vi "padé.vi"(2 "Retardo padé":dbl, 3 "Den":dbl[](array[numeric]), 4 "Num":dbl[](array[numeric])) -> (0 "DEN":dbl[](array[numeric]), 1 "NUM":dbl[](array[numeric]))   [LabVIEW 2019]
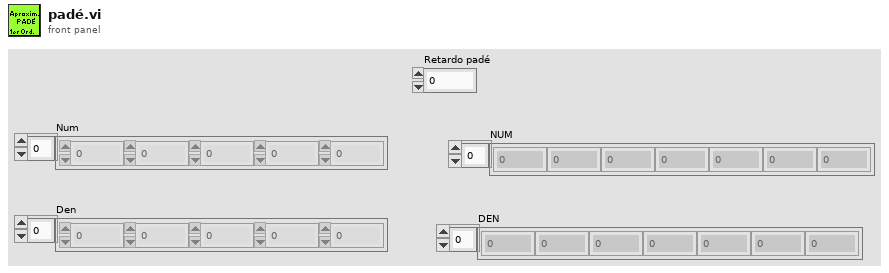
[diagram p1: front panel]
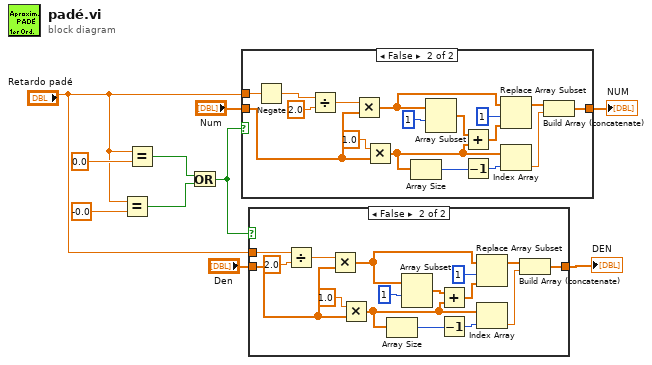
[diagram p0: block diagram]
diagram:
  n1 = Equal?(x="Retardo padé", y=-0.0) -> (x = y?=w7:bool)
  n2 = Equal?(x="Retardo padé", y=0.0) -> (x = y?=w8:bool)
  n3 = Or(x=w8, y=w7) -> (x .or. y?=w2:bool)
  n4 = case shown="False" w2 {
    tunnel: "Retardo padé" -> [_ w15]
    tunnel: [w11 w13] -> w4
    tunnel: "Num" -> [w11 w12]
    frame True {
    }
    frame False {
      n5 = Negate(x=w15) -> (-x=w14:dbl)
      n6 = Divide(x=w14, y=2.0) -> (x/y=w16:dbl)
      n7 = Multiply(x=w16, y=w12) -> (x*y=w23:dbl[])
      n8 = Multiply(x=1.0, y=w12) -> (x*y=w22:dbl[])
      n9 = Array Size(array=w22) -> (size(s)=w21:i32)
      n10 = Array Subset(array=w23, index=1) -> (w26:dbl[])  [unwired: 1 in]
      n11 = Add(x=w26, y=w22) -> (x+y=w25:dbl[])
      n12 = Decrement(x=w21) -> (x-1=w20:i32)
      n13 = Replace Array Subset(array=w23, new element=w25, index=1) -> (w19:dbl[])
      n14 = Index Array(array=w22, index=w20) -> (element=w18:dbl)
      n15 = Build Array (concatenate)(w19, w18) -> (w13:dbl[])
    }
  }
  "NUM" <- w4
  n16 = case shown="False" w2 {
    tunnel: "Retardo padé" -> [_ w30]
    tunnel: [w29 w32] -> w3
    tunnel: "Den" -> [w29 w31]
    frame True {
    }
    frame False {
      n17 = Divide(x=w30, y=2.0) -> (x/y=w33:dbl)
      n18 = Multiply(x=w33, y=w31) -> (x*y=w40:dbl[])
      n19 = Multiply(x=1.0, y=w31) -> (x*y=w39:dbl[])
      n20 = Array Size(array=w39) -> (size(s)=w38:i32)
      n21 = Array Subset(array=w40, index=1) -> (w43:dbl[])  [unwired: 1 in]
      n22 = Add(x=w43, y=w39) -> (x+y=w42:dbl[])
      n23 = Decrement(x=w38) -> (x-1=w37:i32)
      n24 = Replace Array Subset(array=w40, new element=w42, index=1) -> (w36:dbl[])
      n25 = Index Array(array=w39, index=w37) -> (element=w35:dbl)
      n26 = Build Array (concatenate)(w36, w35) -> (w32:dbl[])
    }
  }
  "DEN" <- w3
